vi "checkString.vi"(0 "String":string) -> (1 "String Out":string, 2 "TRUE OR FALSE":bool)   [LabVIEW 2017]
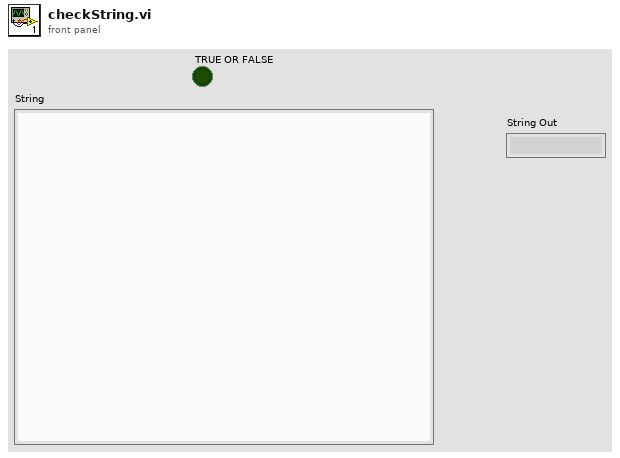
[diagram p1: front panel]
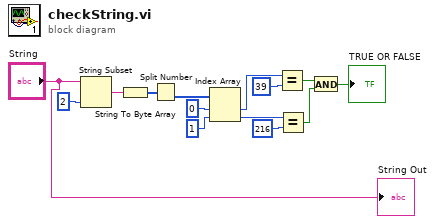
[diagram p0: block diagram]
diagram:
  n1 = String Subset(string="String", length (rest)=2 ("length (rest)")) -> (substring=w13:string)  [unwired: 1 in]
  n2 = String To Byte Array(string=w13) -> (unsigned byte array=w12:u8[])
  n3 = Split Number(x=w12) -> (lo(x)=w11:u8[])  [unwired: 1 out]
  n4 = Index Array(array=w11, index #1=0 ("index"), index #2=1 ("index")) -> (element #1=w7:u8, element #2=w6:u8)
  n5 = Equal?(x=w7, y=u8 39) -> (x = y?=w8:bool)
  n6 = Equal?(x=w6, y=u8 216) -> (x = y?=w3:bool)
  n7 = And(x=w8, y=w3) -> (x .and. y?=→"TRUE OR FALSE":bool)
  "String Out" <- "String"
